vi "picoquant_get_count_rates.vi"(8 "error in (no error)":errorcluster, 11 "picoharp in":refnum<class "picoharp.lvclass">) -> (0 "error out":errorcluster, 2 "count_rates":T1, 3 "picoharp out":refnum<class "picoharp.lvclass">)   [LabVIEW 2015, in "picoharp.lvclass"]
uses:
  picoharp.lvclass
  Hydraharp/hydraharp/hydraharp_count_rates.ctl
  picoharp.lvclass/picoharp.ctl
  phlib.dll
panel:
  out "get_counts_error":i32
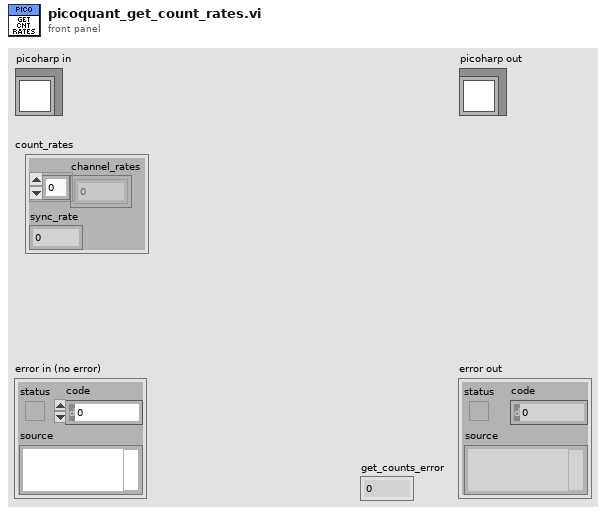
[diagram p1: front panel]
types:
  T1 = typedef "hydraharp_count_rates.ctl" = cluster{"channel_rates":i32[], "sync_rate":i32}
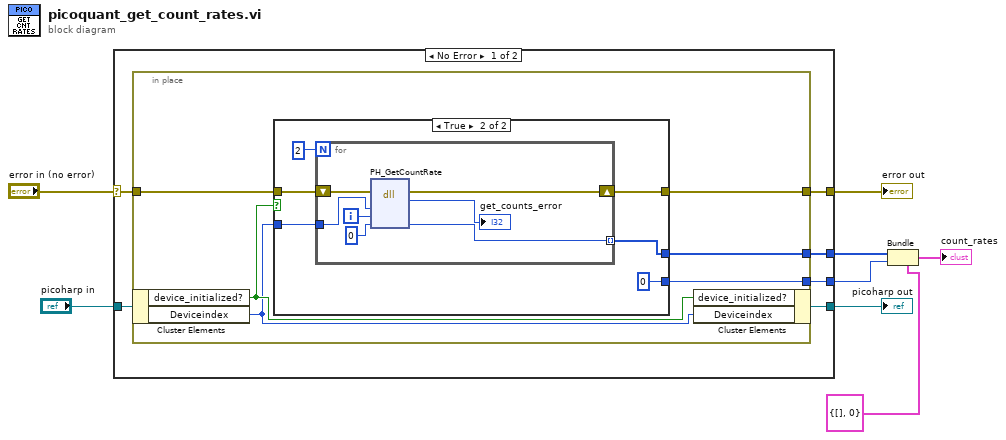
[diagram p0: block diagram]
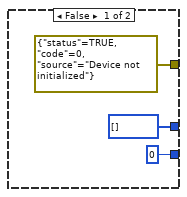
[diagram p2: hidden frame]
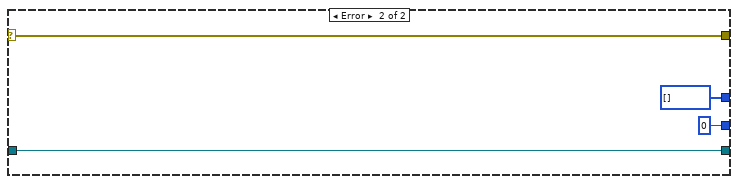
[diagram p3: hidden frame]
diagram:
  n1 = case shown="No Error" "error in (no error)" {
    selector: "error in (no error)" -> [w13 w40]
    tunnel: [w12 w40] -> w5
    tunnel: [w10 w39] -> w2
    tunnel: "picoharp in" -> [w14 w39]
    tunnel: [w11 i32[] []] -> w8
    tunnel: [w9 0 ("rate")] -> w7
    frame No Error {
      n2 = in-place {
        in-place-border: w13 -> [w19]
        in-place-border: [w17] -> w12
        in-place-border: [w16] -> w11
        in-place-border: [w15] -> w9
        n3 = in-place-cluster #1(w14) -> ("device_initialized?"=w20:bool, "Deviceindex"=w18:i32)
        n4 = case shown="True" w20 {
          tunnel: w19 -> [_ w25]
          tunnel: w18 -> [_ w28]
          tunnel: [i32[] [] w27] -> w16
          tunnel: [0 ("rate") 0 ("rate")] -> w15
          tunnel: [errorcluster {"status"=TRUE, "code"=0, "source"="Device not initialized"} ("error out") w26] -> w17
          frame False {
          }
          frame True {
            n5 = for {
              N: 2 -> [_]
              shift-right: [w35] -> w26
              shift-left: w25 -> [w36]
              tunnel: w28 -> [w34]
              tunnel: [w31] -> w27 mode=indexing
              i -> [w33]
              n6 = dll-call lib="phlib.dll" fn="PH_GetCountRate" label="pH_GetCountRate"(error in=w36, "devidx"=w34, "channel"=w33, "rate"=0) -> (error out=w35:errorcluster, "return type"=→"get_counts_error":i32, "rate"=w31:i32)  [unwired: 4 in, 1 out]
            }
          }
        }
        n7 = in-place-cluster #1("device_initialized?"=w20, "Deviceindex"=w18) -> (w10:refnum<class "picoharp.lvclass">)
      }
    }
    frame Error {
    }
  }
  "error out" <- w5
  "picoharp out" <- w2
  n8 = Bundle(cluster=T1 {"channel_rates"=[], "sync_rate"=0} ("output cluster"), "channel_rates"=w8, "sync_rate"=w7) -> (→"count_rates":T1)
